vi "random_sound.vi"() -> ()   [LabVIEW 2018]
panel:
  in  "error in":errorcluster
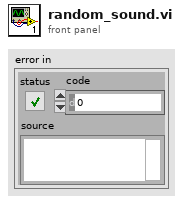
[diagram p1: front panel]
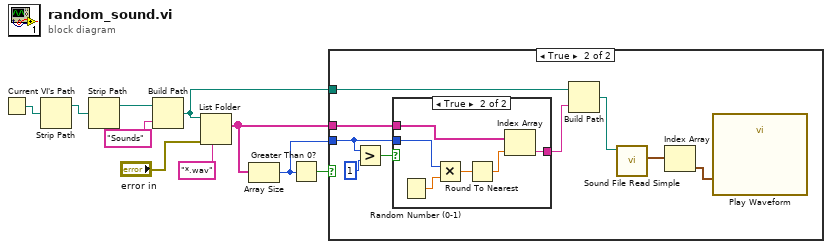
[diagram p0: block diagram]
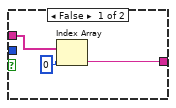
[diagram p3: hidden frame]
diagram:
  n1 = Current VI's Path() -> (path=w10:path)
  n2 = Strip Path(path=w10) -> (stripped path=w3:path)  [unwired: 1 out]
  n3 = Strip Path(path=w3) -> (stripped path=w2:path)  [unwired: 1 out]
  n4 = Build Path(base path=w2, name or relative path="Sounds") -> (appended path=w4:path)
  n5 = List Folder(path=w4, pattern="*.wav", error in="error in") -> (filenames=w5:string[])  [unwired: 1 in, 3 out]
  n6 = Array Size(array=w5) -> (size(s)=w6:i32)
  n7 = Greater Than 0?(x=w6) -> (x > 0?=w7:bool)
  n8 = case shown="True" w7 {
    tunnel: w6 -> [_ w17]
    tunnel: w5 -> [_ w16]
    tunnel: w4 -> [_ w15]
    frame False {
    }
    frame True {
      n9 = Greater?(x=w17, y=1) -> (0:w18:bool)
      n10 = case shown="True" w18 {
        tunnel: w17 -> [_ w27]
        tunnel: w16 -> [w22 w24]
        tunnel: [w20 w23] -> w14
        frame False {
          n11 = Index Array(array=w22, index=0) -> (element=w20:string)
        }
        frame True {
          n12 = Random Number (0-1)() -> (number: 0 to 1=w28:dbl)
          n13 = Multiply(x=w27, y=w28) -> (x*y=w26:dbl)
          n14 = Round To Nearest(number=w26) -> (nearest integer value=w25:dbl)
          n15 = Index Array(array=w24, index=w25) -> (element=w23:string)
        }
      }
      n16 = Build Path(base path=w15, name or relative path=w14) -> (appended path=w13:path)
      n17 = call <vilib>:"Sound File Read Simple.vi"("path"=w13) -> ("data"=w12:waveform(dbl)[])  [unwired: 7 in, 3 out]
      n18 = Index Array(array=w12) -> (element=w11:waveform(dbl))  [unwired: 1 in]
      n19 = call "Play Waveform"("Data"=w11) -> ()  [unwired: 18 in, 1 out]
    }
  }
